vi "CH2_Tx.vi"() -> ()   [LabVIEW 2018]
uses:
  Stream/Stream.lvclass
  RxTx/RxTx.lvclass
panel:
  in  "RxTx.lvclass":refnum<class "RxTx.lvclass">
  in  "Stream.lvclass":refnum<class "Stream.lvclass">
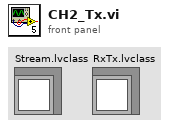
[diagram p1: front panel]
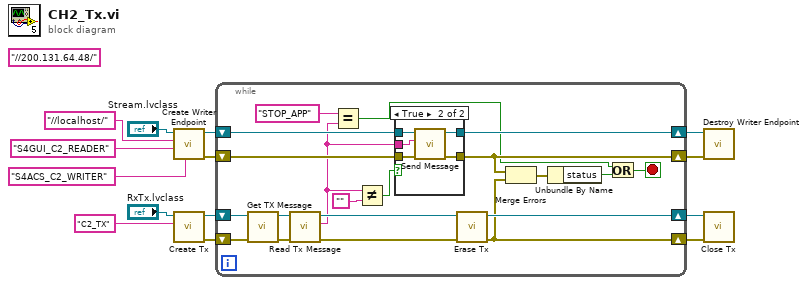
[diagram p0: block diagram]
diagram:
  (unwired) "//200.131.64.48/" ("Reader Name")
  n1 = call "Create Writer Endpoint.vi"("writer name"="S4ACS_C2_WRITER" ("reader name"), "reader name"="S4GUI_C2_READER", "IP"="//localhost/" ("Reader Name"), "Stream in"="Stream.lvclass") -> ("error out"=w6:errorcluster, "Stream out"=w8:refnum<class "Stream.lvclass">)  [unwired: 6 in]
  n2 = call "Create Tx.vi"("Writer Name"="C2_TX" ("Reader Name"), "RxTx in"="RxTx.lvclass") -> ("error out"=w12:errorcluster, "RxTx out"=w13:refnum<class "RxTx.lvclass">)  [unwired: 8 in]
  n3 = while {
    shift-right: [w27] -> w4
    shift-left: w6 -> [w29]
    shift-right: [w28] -> w14
    shift-left: w8 -> [w30]
    shift-right: [w22] -> w9
    shift-left: w12 -> [w31]
    shift-right: [w24] -> w10
    shift-left: w13 -> [w32]
    stop <- w19 stop-if-true
    n4 = call "Get TX Message.vi"("error in (no error)"=w31, "RxTx in"=w32) -> ("error out"=w33:errorcluster, "RxTx out"=w15:refnum<class "RxTx.lvclass">)  [unwired: 8 in]
    n5 = call "Read Tx Message.vi"("error in (no error)"=w33, "RxTx in"=w15) -> ("error out"=w23:errorcluster, "Tx Message"=w16:string, "RxTx out"=w25:refnum<class "RxTx.lvclass">)  [unwired: 7 in]
    n6 = Equal?(x="STOP_APP", y=w16) -> (x = y?=w21:bool)
    n7 = Not Equal?(x=w16, y="") -> (x != y?=w17:bool)
    n8 = case shown="True" w17 {
      tunnel: w30 -> [w36 w41]
      tunnel: w29 -> [w35 w40]
      tunnel: [w36 w39] -> w28
      tunnel: w16 -> [_ w38]
      tunnel: [w35 w37] -> w27
      frame False {
      }
      frame True {
        n9 = call "Send Message.vi"("error in (no error)"=w40, "Message"=w38, "Stream in"=w41) -> ("error out"=w37:errorcluster, "Stream out"=w39:refnum<class "Stream.lvclass">)  [unwired: 7 in]
      }
    }
    n10 = call "Erase Tx.vi"("error in (no error)"=w23, "RxTx in"=w25) -> ("error out"=w22:errorcluster, "RxTx out"=w24:refnum<class "RxTx.lvclass">)  [unwired: 8 in]
    n11 = Merge Errors(w27, w22) -> (w34:errorcluster)
    n12 = Unbundle By Name(w34) -> ("status"=w20:bool)
    n13 = Or(x=w21, y=w20) -> (x .or. y?=w19:bool)
  }
  n14 = call "Destroy Writer Endpoint.vi"("error in (no error)"=w4, "Stream in"=w14) -> ()  [unwired: 8 in, 2 out]
  n15 = call "Close Tx.vi"("error in (no error)"=w9, "RxTx in"=w10) -> ()  [unwired: 8 in, 2 out]
